vi "Engine In - PFI - Sensors.vi"(0 "dt [sec]":sgl, 1 "ADCombo.Voltage [V]":sgl[](array[numeric]), 2 "ADCombo.Resistance [Ohm]":sgl[](array[numeric])) -> (7 "Fuel Temp [C]":sgl, 8 "TDKBattV":sgl format="%0.2f", 9 "MAT [C]":sgl format="%0.2f", 10 "12VPulsBattV":sgl format="%0.2f", 12 "5VPulsBattV":sgl format="%0.2f", 13 "IAT [C]":sgl, 14 "Fuel Pressure [kPa]":sgl format="%0.2f", 15 "ECT [C]":sgl format="%0.2f", 16 "Barometric Air Pressure [kPa]":sgl, 18 "CAC Outlet Pressure [kPa]":sgl, 20 "MAP [kPa]":sgl format="%0.2f", 23 "Oil Pressure [kPa]":sgl, 24 "MAF [kg/hr]":sgl format="%0.2f", 26 "Pedal [%]":sgl format="%0.2f")   [LabVIEW 2015, in "ECS-RT.lvlib"]
uses:
  ECS-RT.lvlib
  <vilib>/ptbypt/NI_PtbyPt.lvlib
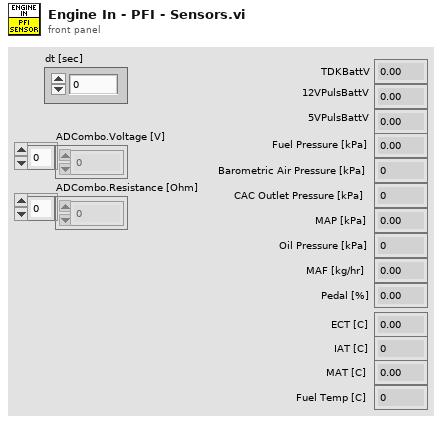
[diagram p1: front panel]
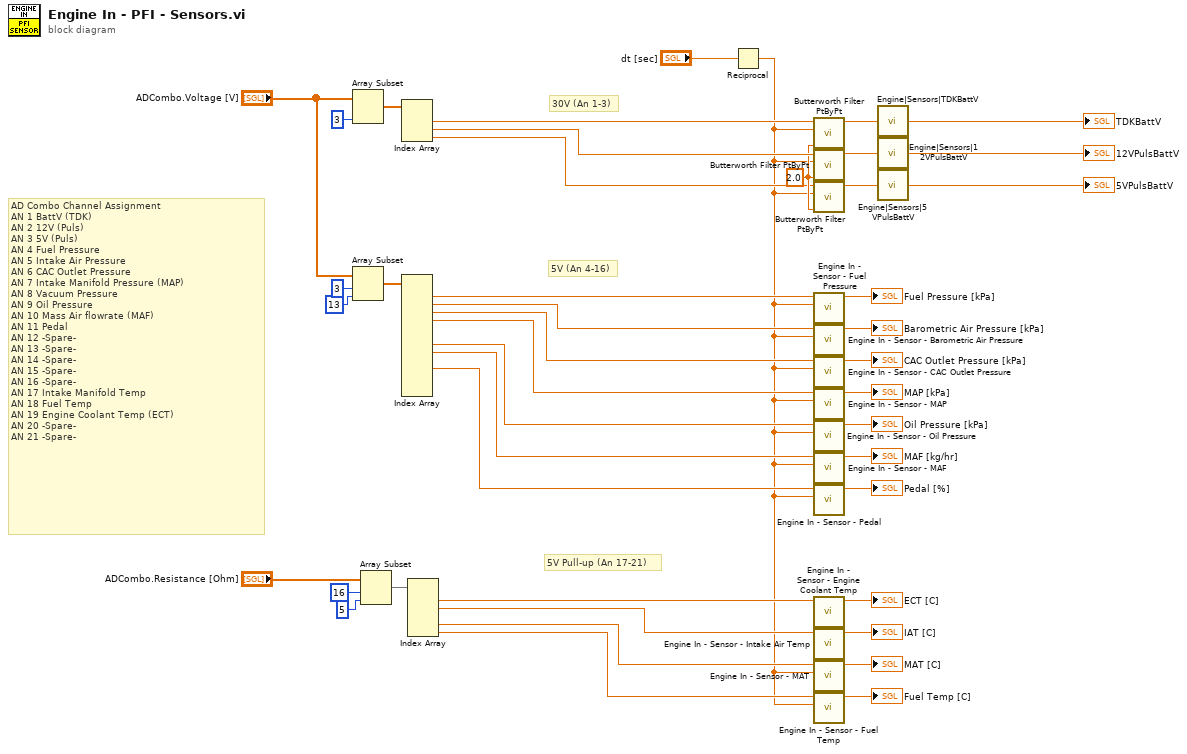
[diagram p0: block diagram]
diagram:
  w34 = 2.0 ("low cutoff freq: fl")
  # "5V Pull-up (An 17-21)"
  # "5V (An 4-16)"
  # "30V (An 1-3)"
  # "AD Combo Channel Assignment\nAN\t1\tBattV (TDK)\nAN\t2\t12V (Puls)\nAN\t3\t5V (Puls)\nAN\t4\tFuel Pressure\nAN\t5\tIntake Air Pressure\nAN\t6\tCAC Outlet Pressure\nAN\t7\tIntake Manifold Pressure (MAP)\nAN\t8\tVacuum Pressure\nAN\t9\tOil Pressure\nAN\t10\tMass Air flowrate (MAF)\nAN\t11\tPedal\nAN 12 -Spare-\nAN\t13\t-Spare-\nAN\t14\t-Spare-\nAN\t15\t-Spare-\nAN\t16\t-Spare-\nAN\t17\tIntake Manifold Temp\nAN\t18\tFuel Temp\nAN\t19\tEngine Coolant Temp (ECT)\nAN 20 -Spare-\nAN\t21\t-Spare-"
  n1 = Array Subset(array="ADCombo.Voltage [V]", length=3) -> (w28:sgl[])  [unwired: 1 in]
  n2 = Array Subset(array="ADCombo.Voltage [V]", index=3, length=13) -> (w27:sgl[])
  n3 = Array Subset(array="ADCombo.Resistance [Ohm]", index=16, length=5) -> (w26:sgl[])
  n4 = Index Array(array=w28) -> (element #1=w37:sgl, element #2=w36:sgl, element #3=w17:sgl)  [unwired: 3 in]
  n5 = Index Array(array=w27) -> (element #1=w14:sgl, element #2=w2:sgl, element #3=w13:sgl, element #4=w12:sgl, element #7=w10:sgl, element #8=w9:sgl, element #10=w11:sgl)  [unwired: 13 in, 6 out]
  n6 = Index Array(array=w26) -> (element #1=w8:sgl, element #2=w4:sgl, element #4=w6:sgl, element #5=w7:sgl)  [unwired: 5 in, 1 out]
  n7 = Reciprocal(x="dt [sec]") -> (1/x=w1:sgl)
  n8 = call <vilib>:"Butterworth Filter PtByPt.vi"("low cutoff freq: fl"=w34, "sampling freq: fs"=w1, "x"=w37) -> ("Filtered x"=w32:dbl)  [unwired: 4 in, 3 out]
  "TDKBattV" <- w32
  n9 = call <vilib>:"Butterworth Filter PtByPt.vi"("low cutoff freq: fl"=w34, "sampling freq: fs"=w1, "x"=w36) -> ("Filtered x"=w31:dbl)  [unwired: 4 in, 3 out]
  "12VPulsBattV" <- w31
  n10 = call <vilib>:"Butterworth Filter PtByPt.vi"("low cutoff freq: fl"=w34, "sampling freq: fs"=w1, "x"=w17) -> ("Filtered x"=w30:dbl)  [unwired: 4 in, 3 out]
  "5VPulsBattV" <- w30
  n11 = call "Engine In - Sensor - Fuel Pressure.vi"("Loop Freq (Hz)"=w1, "Fuel Pressure [V]"=w14) -> ("Fuel Pressure [bar]"=→"Fuel Pressure [kPa]":sgl)  [unwired: 9 in]
  n12 = call "Engine In - Sensor - Barometric Air Pressure.vi"("Loop Freq (Hz)"=w1, "Barometric Air Pressure [V]"=w2) -> ("Barometric Air Pressure [kPa]"=→"Barometric Air Pressure [kPa]":sgl)  [unwired: 9 in]
  n13 = call "Engine In - Sensor - CAC Outlet Pressure.vi"("Loop Freq (Hz)"=w1, "CAC Outlet Pressure [V]"=w13) -> ("CAC Outlet Pressure [kPa]"=→"CAC Outlet Pressure [kPa]":sgl)  [unwired: 9 in]
  n14 = call "Engine In - Sensor - MAP.vi"("Loop Freq (Hz)"=w1, "Raw Intake Manifold Pressure [V]"=w12) -> ("Intake Manifold Pressure [kPa]"=→"MAP [kPa]":sgl)  [unwired: 9 in]
  n15 = call "Engine In - Sensor - Oil Pressure.vi"("Loop Freq (Hz)"=w1, "Oil Pressure [V]"=w10) -> ("Oil Pressure [kPa]"=→"Oil Pressure [kPa]":sgl)  [unwired: 9 in]
  n16 = call "Engine In - Sensor - MAF.vi"("Loop Freq (Hz)"=w1, "MAF [V]"=w9) -> ("MAF [kg/hr]"=→"MAF [kg/hr]":sgl)  [unwired: 9 in]
  n17 = call "Engine In - Sensor - Pedal.vi"("Loop Freq (Hz)"=w1, "Pedal [V]"=w11) -> ("Pedal [%]"=→"Pedal [%]":sgl)  [unwired: 9 in]
  n18 = call "Engine In - Sensor - Engine Coolant Temp.vi"("Engine Coolant Temp Raw [Ohm]"=w8) -> ("Engine Coolant Temp [C]"=→"ECT [C]":sgl)  [unwired: 10 in]
  n19 = call "Engine In - Sensor - Intake Air Temp.vi"("Intake Air Temp Raw [Ohm]"=w4) -> ("Intake Air Temp [C]"=→"IAT [C]":sgl)  [unwired: 10 in]
  n20 = call "Engine In - Sensor - MAT.vi"("Loop Freq [Hz]"=w1, "Raw Intake Manifold Temp [Ohm]"=w6) -> ("Intake Manifold Temp [C]"=→"MAT [C]":sgl)  [unwired: 9 in]
  n21 = call "Engine In - Sensor - Fuel Temp.vi"("Loop Freq [Hz]"=w1, "Fuel Temp Raw [Ohm]"=w7) -> ("Fuel Temp [C]"=→"Fuel Temp [C]":sgl)  [unwired: 9 in]
  n22 = call "Engine|Sensors|TDKBattV"("Value"=w32) -> ()
  n23 = call "Engine|Sensors|12VPulsBattV"("Value"=w31) -> ()
  n24 = call "Engine|Sensors|5VPulsBattV"("Value"=w30) -> ()
